vi "Get State.vi"(8 "error in (no error)":errorcluster, 10 "Cycle count":i32, 11 "Response Synchronizer in":refnum<class "Response Synchronizer.lvclass">) -> (0 "error out":errorcluster, 1 "Awaiting results":bool, 2 "Result ready":bool, 3 "Response Synchronizer out":refnum<class "Response Synchronizer.lvclass">, 4 "Cycle counters":i32[](array[numeric]), 5 "Results":refnum<class "Acquired Result.lvclass">[](array[class]), 6 "Measurement counters":i32[](array[numeric]))   [LabVIEW 2024, in "Response Synchronizer.lvclass"]
uses:
  Response Synchronizer.lvclass
  NHMFL_Core/Libraries/Instruments/Results/Acquired Result/Acquired Result.lvclass
  Response Synchronizer.lvclass/Response Synchronizer.ctl
panel:
  out "call chain":string[](array[string])
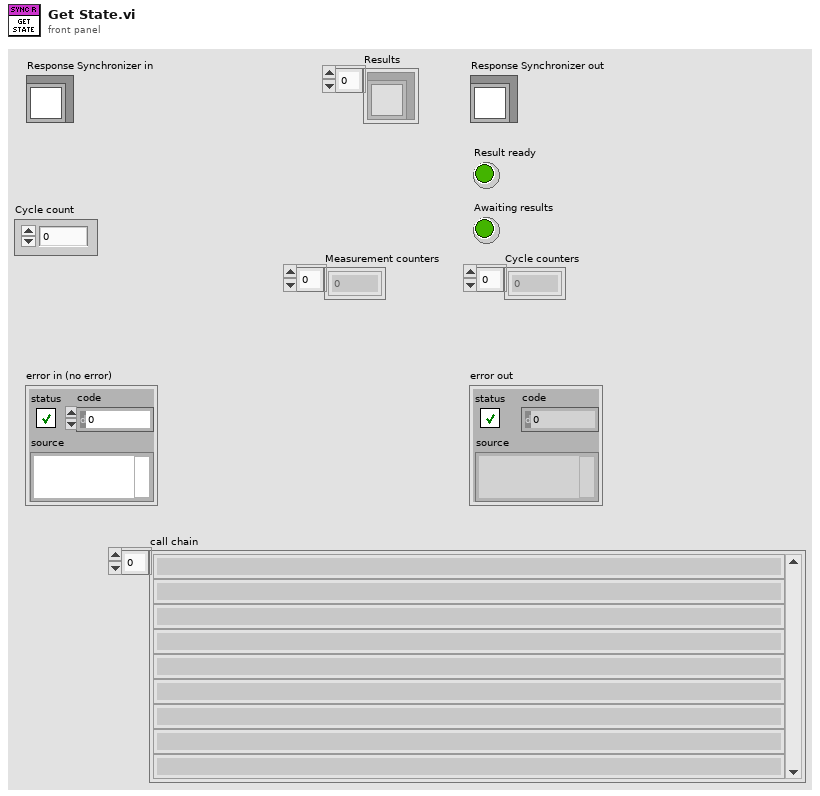
[diagram p1: front panel]
types:
  T1 = map{cluster{"Accessors:Sender":string, "Accessors:Cycle count":i32}, refnum<class "Acquired Result.lvclass">}
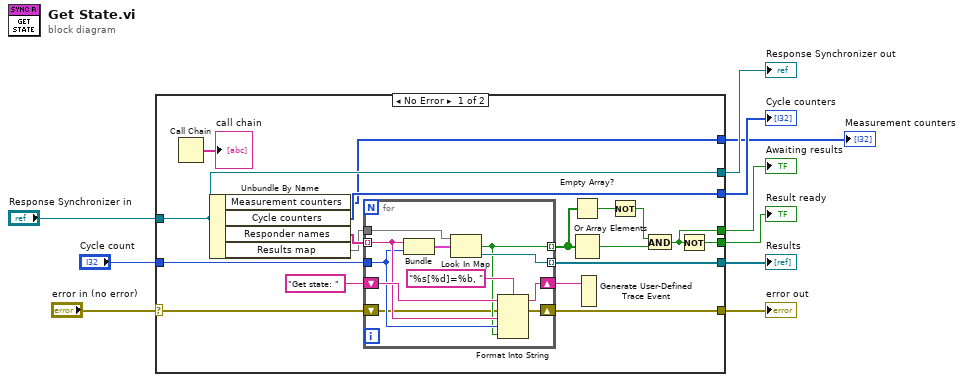
[diagram p0: block diagram]
diagram:
  n1 = case shown="No Error" "error in (no error)" {
    selector: "error in (no error)" -> [w14 w41]
    tunnel: [w13 w41] -> w9
    tunnel: [w25 w40] -> w7
    tunnel: "Response Synchronizer in" -> [w25 w40]
    tunnel: [w19 _] -> w6
    tunnel: [w18 _] -> w5
    tunnel: [w24 _] -> w4
    tunnel: "Cycle count" -> [w22 _]
    tunnel: [w17 _] -> w2
    tunnel: [w11 _] -> w1
    frame No Error {
      n2 = Call Chain() -> (call chain=→"call chain":string[])
      n3 = Unbundle By Name(w25) -> ("Measurement counters"=w11:i32[], "Cycle counters"=w24:i32[], "Responder names"=w23:string[], "Results map"=w21:T1)
      n4 = for {
        tunnel: w23 -> [w35] mode=indexing
        tunnel: w22 -> [w34]
        tunnel: w21 -> [w39]
        tunnel: [w32] -> w20 mode=indexing
        tunnel: [w37] -> w17 mode=indexing
        shift-right: [w31] -> w15
        shift-left: "Get state: " ("format string") -> [w36]
        shift-right: [w29] -> w13
        shift-left: w14 -> [w30]
        n5 = Bundle("String"=w35, "Cycle count"=w34) -> (w38:cluster{"String":string, "Cycle count":i32})  [unwired: 1 in]
        n6 = Look In Map(map=w39, key=w38) -> (key not found?=w32:bool, value=w37:refnum<class "Acquired Result.lvclass">)  [unwired: 1 in]
        n7 = Format Into String(format string="%s[%d]=%b, ", initial string=w36, error in=w30, w35, w34, w32) -> (resulting string=w31:string, error out=w29:errorcluster)
      }
      n8 = Empty Array?(array=w20) -> (empty?=w27:bool)
      n9 = Or Array Elements(Boolean array=w20) -> (logical OR=w28:bool)
      n10 = Generate User-Defined Trace Event(2:w15) -> ()  [unwired: 1 in]
      n11 = Not(x=w27) -> (.not. x?=w26:bool)
      n12 = And(x=w26, y=w28) -> (x .and. y?=w19:bool)
      n13 = Not(x=w19) -> (.not. x?=w18:bool)
    }
    frame Error {
    }
  }
  "error out" <- w9
  "Response Synchronizer out" <- w7
  "Result ready" <- w5
  "Awaiting results" <- w6
  "Cycle counters" <- w4
  "Results" <- w2
  "Measurement counters" <- w1
